vi "sub_Text_To_Bitstream.vi"(9 "Packet\nMessage Length (bits)":i32, 11 "text":string) -> (1 "File Length (bits)":i32, 3 "message bitstream":i8[](array[numeric]), 4 "Number of Packets":i32)   [LabVIEW 2013]
panel:
  out "Numeric":dbl
  out "Array":i8[][](array[numeric])
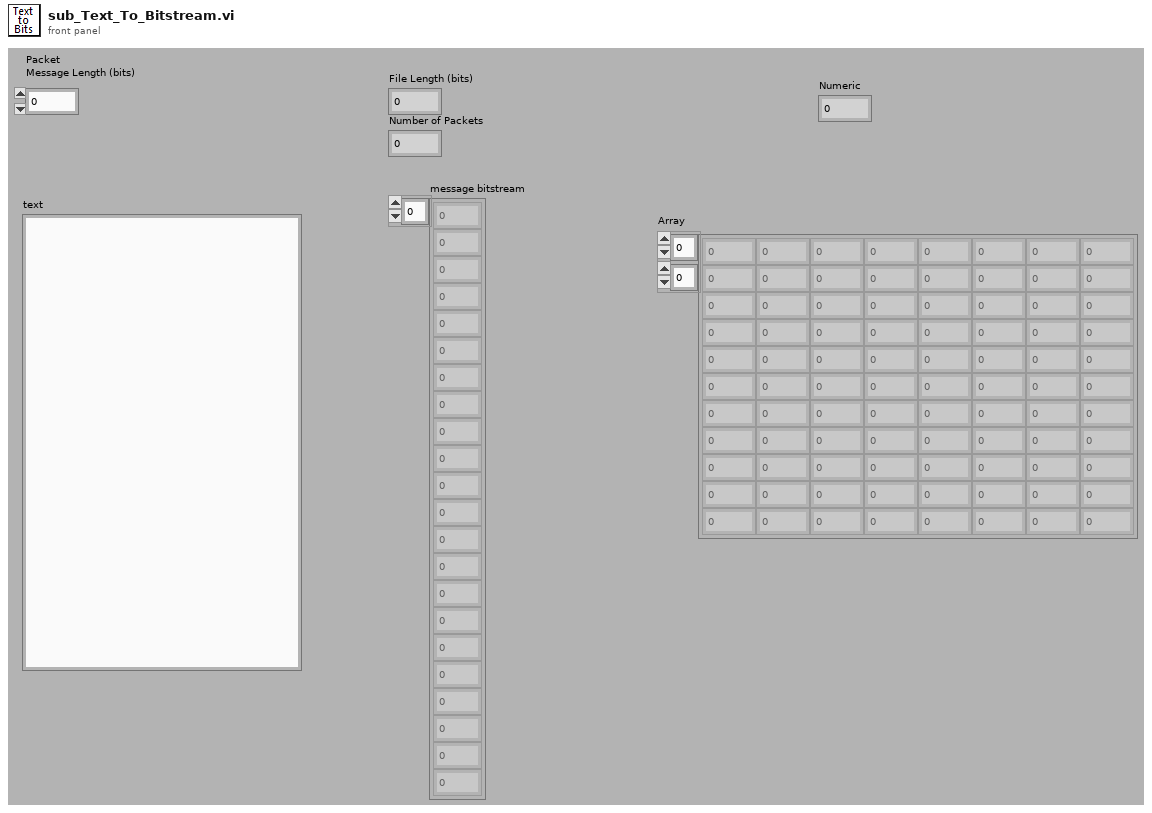
[diagram p1: front panel]
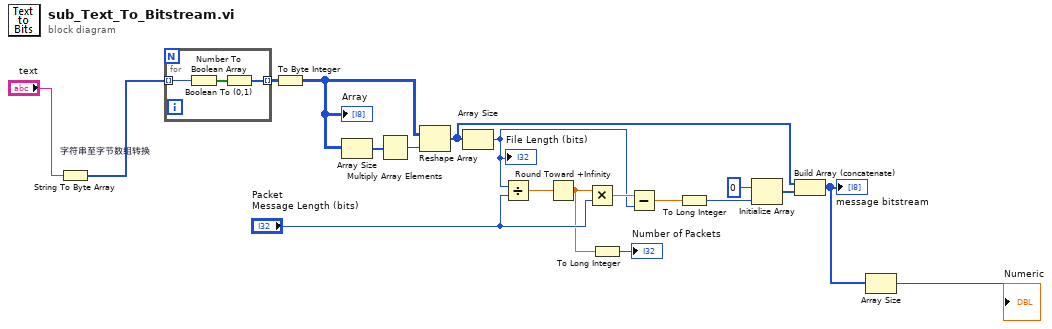
[diagram p0: block diagram]
diagram:
  n1 = String To Byte Array "字符串至字节数组转换"(string="text") -> (unsigned byte array=w18:u8[])
  n2 = for {
    tunnel: w18 -> [w22] mode=indexing
    tunnel: [w20] -> w17 mode=indexing
    n3 = Number To Boolean Array(number=w22) -> (Boolean array=w21:bool[])
    n4 = Boolean To (0,1)(Boolean=w21) -> (0, 1=w20:i16[])
  }
  n5 = To Byte Integer(number=w17) -> (8bit integer=w3:i8[][])
  "Array" <- w3
  n6 = Array Size(array=w3) -> (size(s)=w16:i32[])
  n7 = Multiply Array Elements ("数组元素相乘")(1:w16) -> (0:w15:i32)
  n8 = Reshape Array(w3, w15) -> (w5:i8[])
  n9 = Array Size(array=w5) -> (size(s)=w11:i32)
  "File Length (bits)" <- w11
  n10 = Divide(x=w11, y="Packet\nMessage Length (bits)") -> (x/y=w13:dbl)
  n11 = Round Toward +Infinity(x=w13) -> (ceil(x): smallest int >= x=w8:dbl)
  n12 = Multiply(x=w8, y="Packet\nMessage Length (bits)") -> (x*y=w12:dbl)
  n13 = To Long Integer(number=w8) -> (32bit integer=→"Number of Packets":i32)
  n14 = Subtract(x=w12, y=w11) -> (x-y=w10:dbl)
  n15 = To Long Integer(number=w10) -> (32bit integer=w6:i32)
  n16 = Initialize Array(i8 0 ("element"), w6) -> (w4:i8[])
  n17 = Build Array (concatenate)(w5, w4) -> (w2:i8[])
  "message bitstream" <- w2
  n18 = Array Size(array=w2) -> (size(s)=→"Numeric":i32)
